vi "is a.vi"(8 "error in (no error)":errorcluster, 11 "DMM in":refnum<class "DMM.lvclass">) -> (0 "error out":errorcluster, 2 "is a":string, 3 "DMM out":refnum<class "DMM.lvclass">)   [LabVIEW 2017, in "Hardware.lvlib" / "DMM.lvclass"]
uses:
  DMM.lvclass
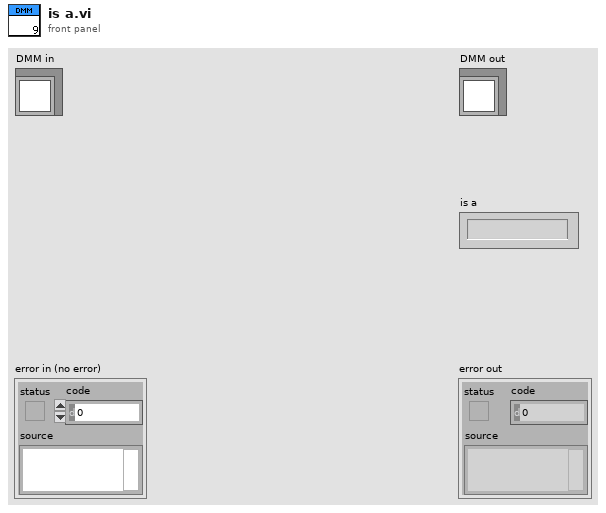
[diagram p1: front panel]
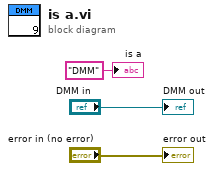
[diagram p0: block diagram]
diagram:
  "error out" <- "error in (no error)"
  "DMM out" <- "DMM in"
  "is a" <- "DMM" ("is a")
